vi "PruebaPAI.vi"() -> ()   [LabVIEW 2024]
uses:
  <vilib>/MakerHub/LINX/Public/Peripherals/Digital/Digital Read 1 Chan.vi
  <vilib>/MakerHub/LINX/Public/Peripherals/Digital/Digital Write 1 Chan.vi
  <vilib>/MakerHub/LINX/Public/Peripherals/Digital/Digital Read N Chans.vi
  <vilib>/MakerHub/LINX/Public/Peripherals/Digital/Digital Write N Chans.vi
  <vilib>/MakerHub/LINX/Private/Local IO/LinxDigitalRead.vi
  <vilib>/MakerHub/LINX/Public/Utilities/Check Channel.vi
  <vilib>/MakerHub/LINX/Private/Local IO/LinxDigitalWrite.vi
  <vilib>/MakerHub/LINX/Public/Utilities/Open Serial.vi
  <vilib>/MakerHub/LINX/Private/Utilties/Generate Error.vi
  <vilib>/MakerHub/LINX/LMH-LINX.lvlib
panel:
  in  "Detener":bool
  out "Pin6":dbl
  out "Pin5":dbl
  out "Pin4":dbl
  out "Pin3":dbl
  out "Pin2":dbl
  in  "Puerto Serial":refnum<visa-resource-name>="N/A"
  out "Contenido":dbl
  out "Led 5":bool
  out "Led 4":bool
  out "Led 3":bool
  in  "Secuencia":dbl
  out "Led 2":bool
  out "Led 1":bool
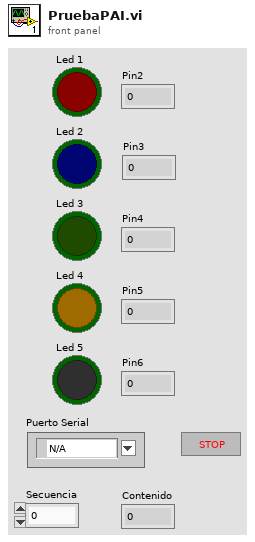
[diagram p1: front panel]
types:
  T1 = typedef "LMH-LINX.lvlib/LINX Ref.ctl" = cluster{"IO":T2, "Interface":T3, "LINX Device Config":T4}
  T2 = typedef "LMH-LINX.lvlib/Platform.ctl" = enum16{"Remote", "Local"}
  T3 = typedef "LMH-LINX.lvlib/Interface.ctl" = enum16{"Serial", "TCP"}
  T4 = typedef "LMH-LINX.lvlib/Device.lvlib/LINX Device Config.ctl" = cluster{"Interface":T3, "COM Port":refnum<visa-resource-name>, "TCP Configuration":T5, "Device Family":u8, "Device ID":u8, "Device Name":string, "TCP Ref":refnum<k5>, "Channels":T6}
  T5 = typedef "LMH-LINX.lvlib/Device.lvlib/TCP Config.ctl" = cluster{"IP Address":string, "Port":u16}
  T6 = typedef "LMH-LINX.lvlib/Channels.ctl" = cluster{"DI":u8[], "DO":u8[], "AI":u8[], "AO":u8[], "PWM":u8[], "QE":u8[], "UART":u8[], "I2C 2":u8[], "SPI":u8[], "CAN":u8[], "Servo":u8[], "AI Ref (V)":dbl, "AI Resolution (Bits)":u8, "AO Ref (V)":dbl, "AO Resolution (Bits)":u8}
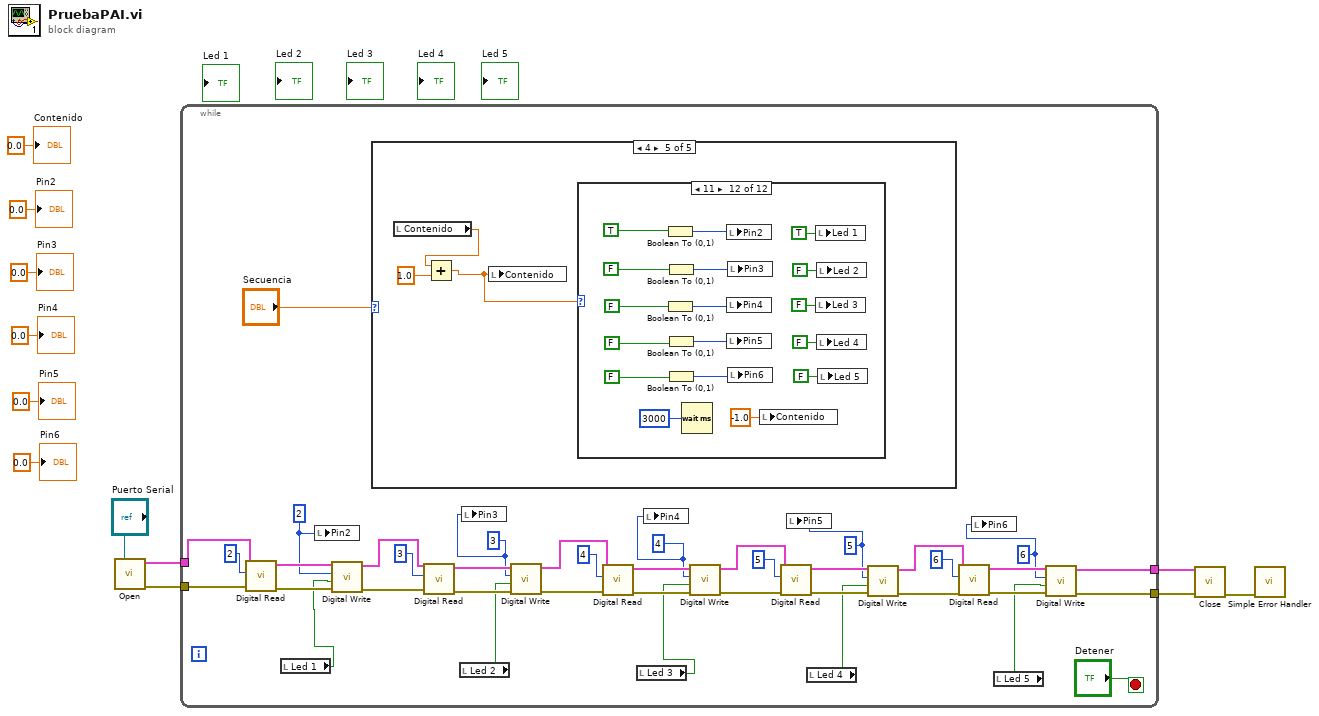
[diagram p0: block diagram]
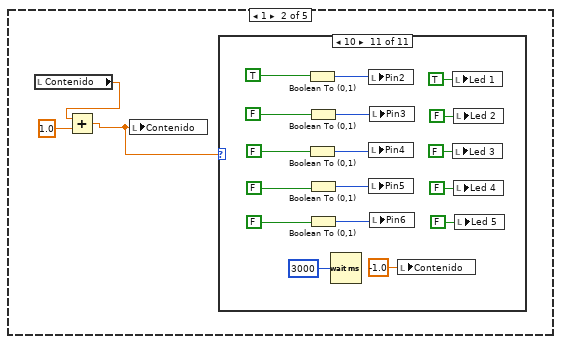
[diagram p3: hidden frame]
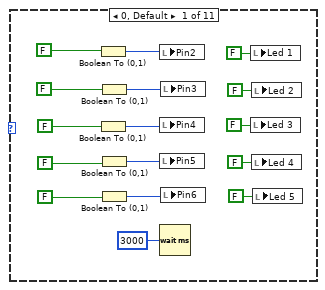
[diagram p4: hidden frame]
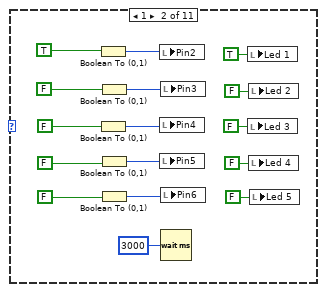
[diagram p5: hidden frame]
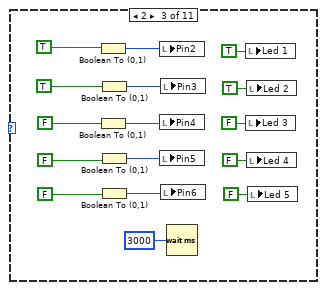
[diagram p6: hidden frame]
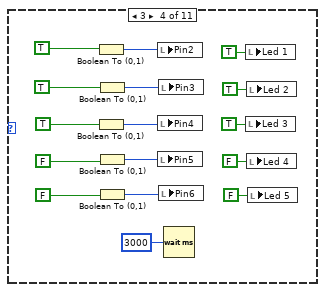
[diagram p7: hidden frame]
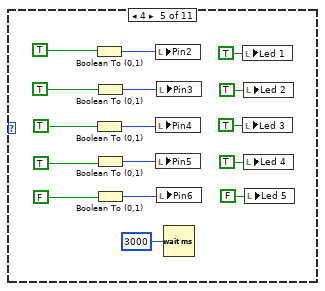
[diagram p8: hidden frame]
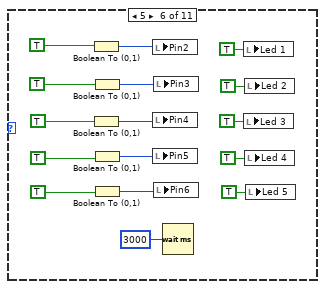
[diagram p9: hidden frame]
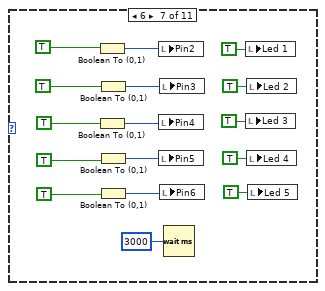
[diagram p10: hidden frame]
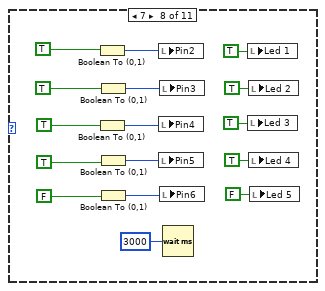
[diagram p11: hidden frame]
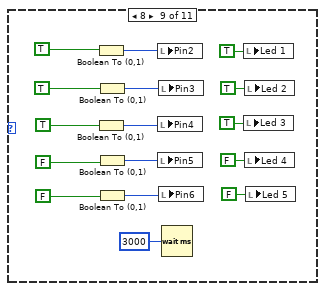
[diagram p12: hidden frame]
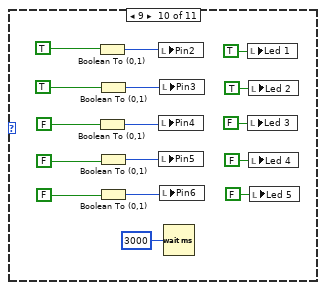
[diagram p13: hidden frame]
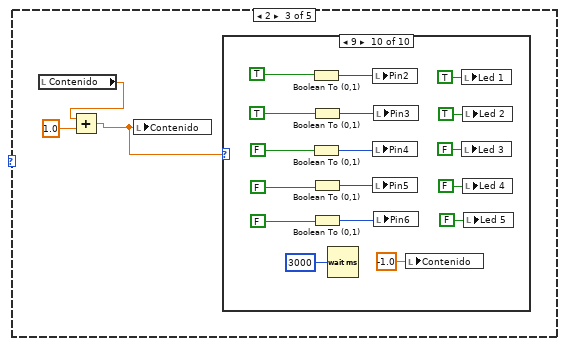
[diagram p14: hidden frame]
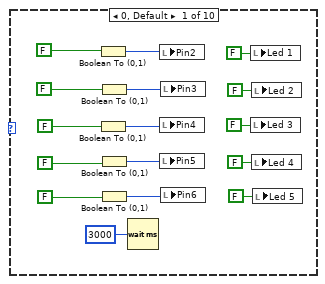
[diagram p15: hidden frame]
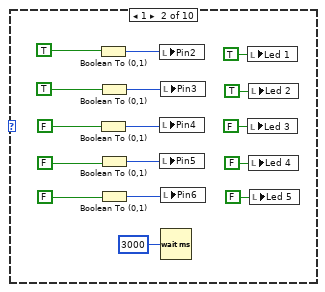
[diagram p16: hidden frame]
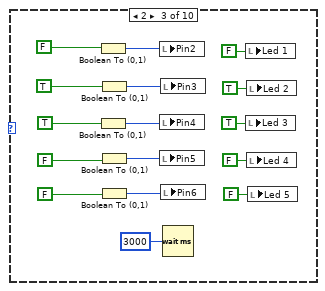
[diagram p17: hidden frame]
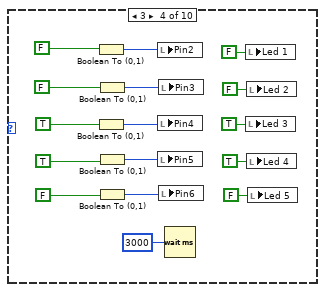
[diagram p18: hidden frame]
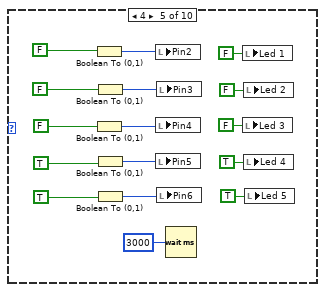
[diagram p19: hidden frame]
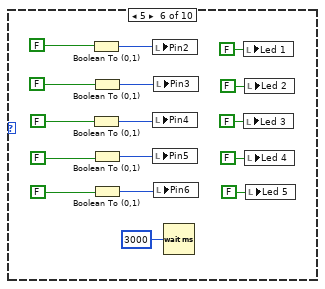
[diagram p20: hidden frame]
diagram:
  n1 = call-poly <vilib>:"Open.vi"("Serial Port"="Puerto Serial") -> ("Error Out"=w1:errorcluster, "LINX Resource"=w2:T1)  [unwired: 8 in, 1 out]
  n2 = while {
    tunnel: [w18] -> w4
    tunnel: [w17] -> w3
    tunnel: w2 -> [w16]
    tunnel: w1 -> [w15]
    stop <- "Detener" stop-if-true
    w19 = u8 6 ("DO Channel")
    w22 = u8 5 ("DO Channel")
    w23 = u8 4 ("DO Channel")
    w28 = u8 3 ("DO Channel")
    w26 = u8 2 ("DO Channel")
    n3 = call-poly <vilib>:"Digital Read.vi"("Error In"=w15, "DI Channel"=u8 2, "LINX Resource"=w16) -> ("Error Out"=w37:errorcluster, "LINX Resource"=w46:T1)  [unwired: 6 in, 1 out]
    n4 = local read "Led 1"() -> (w27:bool)
    n5 = local write "Pin2"(w26) -> ()
    n6 = call-poly <vilib>:"Digital Write.vi"("Error In"=w37, "Output Value"=w27, "DO Channel"=w26, "LINX Resource"=w46) -> ("Error Out"=w36:errorcluster, "LINX Resource"=w45:T1)  [unwired: 6 in]
    n7 = case shown="4" "Secuencia" {
      frame 0, Default {
      }
      frame 1 {
        n8 = local read "Contenido"() -> (w53:dbl)
        n9 = Add(x=w53, y=1.0) -> (x+y=w52:dbl)
        n10 = local write "Contenido"(w52) -> ()
        n11 = case shown="10" w52 {
          frame 0, Default {
            n12 = Boolean To (0,1)(Boolean=FALSE) -> (0, 1=w70:i16)
            n13 = Boolean To (0,1)(Boolean=FALSE) -> (0, 1=w68:i16)
            n14 = Boolean To (0,1)(Boolean=FALSE) -> (0, 1=w69:i16)
            n15 = Boolean To (0,1)(Boolean=FALSE) -> (0, 1=w67:i16)
            n16 = Boolean To (0,1)(Boolean=FALSE) -> (0, 1=w66:i16)
            n17 = local write "Pin2"(w70) -> ()
            n18 = local write "Pin4"(w68) -> ()
            n19 = local write "Pin5"(w67) -> ()
            n20 = Wait (ms)(milliseconds to wait=u32 3000 ("millisecond timer value")) -> ()  [unwired: 1 out]
            n21 = local write "Pin3"(w69) -> ()
            n22 = local write "Pin6"(w66) -> ()
            n23 = local write "Led 1"(FALSE ("Led 1")) -> ()
            n24 = local write "Led 3"(FALSE ("Led 3")) -> ()
            n25 = local write "Led 2"(FALSE ("Led 2")) -> ()
            n26 = local write "Led 4"(FALSE ("Led 4")) -> ()
            n27 = local write "Led 5"(FALSE ("Led 5")) -> ()
          }
          frame 1 {
            n28 = Boolean To (0,1)(Boolean=TRUE) -> (0, 1=w85:i16)
            n29 = Boolean To (0,1)(Boolean=FALSE) -> (0, 1=w81:i16)
            n30 = Boolean To (0,1)(Boolean=FALSE) -> (0, 1=w83:i16)
            n31 = Boolean To (0,1)(Boolean=FALSE) -> (0, 1=w79:i16)
            n32 = Boolean To (0,1)(Boolean=FALSE) -> (0, 1=w77:i16)
            n33 = local write "Pin2"(w85) -> ()
            n34 = local write "Pin4"(w81) -> ()
            n35 = local write "Pin5"(w79) -> ()
            n36 = local write "Pin3"(w83) -> ()
            n37 = local write "Pin6"(w77) -> ()
            n38 = Wait (ms)(milliseconds to wait=u32 3000 ("millisecond timer value")) -> ()  [unwired: 1 out]
            n39 = local write "Led 1"(TRUE ("Led 1")) -> ()
            n40 = local write "Led 3"(FALSE ("Led 3")) -> ()
            n41 = local write "Led 2"(FALSE ("Led 2")) -> ()
            n42 = local write "Led 4"(FALSE ("Led 4")) -> ()
            n43 = local write "Led 5"(FALSE ("Led 5")) -> ()
          }
          frame 2 {
            n44 = Boolean To (0,1)(Boolean=TRUE) -> (0, 1=w102:i16)
            n45 = Boolean To (0,1)(Boolean=FALSE) -> (0, 1=w100:i16)
            n46 = Boolean To (0,1)(Boolean=TRUE) -> (0, 1=w101:i16)
            n47 = Boolean To (0,1)(Boolean=FALSE) -> (0, 1=w99:i16)
            n48 = Boolean To (0,1)(Boolean=FALSE) -> (0, 1=w98:i16)
            n49 = local write "Pin2"(w102) -> ()
            n50 = local write "Pin4"(w100) -> ()
            n51 = local write "Pin5"(w99) -> ()
            n52 = local write "Pin3"(w101) -> ()
            n53 = local write "Pin6"(w98) -> ()
            n54 = Wait (ms)(milliseconds to wait=u32 3000 ("millisecond timer value")) -> ()  [unwired: 1 out]
            n55 = local write "Led 1"(TRUE ("Led 1")) -> ()
            n56 = local write "Led 3"(FALSE ("Led 3")) -> ()
            n57 = local write "Led 2"(TRUE ("Led 2")) -> ()
            n58 = local write "Led 4"(FALSE ("Led 4")) -> ()
            n59 = local write "Led 5"(FALSE ("Led 5")) -> ()
          }
          frame 3 {
            n60 = Boolean To (0,1)(Boolean=TRUE) -> (0, 1=w118:i16)
            n61 = Boolean To (0,1)(Boolean=TRUE) -> (0, 1=w116:i16)
            n62 = Boolean To (0,1)(Boolean=TRUE) -> (0, 1=w117:i16)
            n63 = Boolean To (0,1)(Boolean=FALSE) -> (0, 1=w115:i16)
            n64 = Boolean To (0,1)(Boolean=FALSE) -> (0, 1=w114:i16)
            n65 = local write "Pin2"(w118) -> ()
            n66 = local write "Pin4"(w116) -> ()
            n67 = local write "Pin5"(w115) -> ()
            n68 = local write "Pin3"(w117) -> ()
            n69 = local write "Pin6"(w114) -> ()
            n70 = Wait (ms)(milliseconds to wait=u32 3000 ("millisecond timer value")) -> ()  [unwired: 1 out]
            n71 = local write "Led 1"(TRUE ("Led 1")) -> ()
            n72 = local write "Led 3"(TRUE ("Led 3")) -> ()
            n73 = local write "Led 2"(TRUE ("Led 2")) -> ()
            n74 = local write "Led 4"(FALSE ("Led 4")) -> ()
            n75 = local write "Led 5"(FALSE ("Led 5")) -> ()
          }
          frame 4 {
            n76 = Boolean To (0,1)(Boolean=TRUE) -> (0, 1=w134:i16)
            n77 = Boolean To (0,1)(Boolean=TRUE) -> (0, 1=w132:i16)
            n78 = Boolean To (0,1)(Boolean=TRUE) -> (0, 1=w133:i16)
            n79 = Boolean To (0,1)(Boolean=TRUE) -> (0, 1=w131:i16)
            n80 = Boolean To (0,1)(Boolean=FALSE) -> (0, 1=w130:i16)
            n81 = local write "Pin2"(w134) -> ()
            n82 = local write "Pin4"(w132) -> ()
            n83 = local write "Pin5"(w131) -> ()
            n84 = local write "Pin3"(w133) -> ()
            n85 = local write "Pin6"(w130) -> ()
            n86 = Wait (ms)(milliseconds to wait=u32 3000 ("millisecond timer value")) -> ()  [unwired: 1 out]
            n87 = local write "Led 1"(TRUE ("Led 1")) -> ()
            n88 = local write "Led 3"(TRUE ("Led 3")) -> ()
            n89 = local write "Led 2"(TRUE ("Led 2")) -> ()
            n90 = local write "Led 4"(TRUE ("Led 4")) -> ()
            n91 = local write "Led 5"(FALSE ("Led 5")) -> ()
          }
          frame 5 {
            n92 = Boolean To (0,1)(Boolean=TRUE) -> (0, 1=w150:i16)
            n93 = Boolean To (0,1)(Boolean=TRUE) -> (0, 1=w148:i16)
            n94 = Boolean To (0,1)(Boolean=TRUE) -> (0, 1=w149:i16)
            n95 = Boolean To (0,1)(Boolean=TRUE) -> (0, 1=w147:i16)
            n96 = Boolean To (0,1)(Boolean=TRUE) -> (0, 1=w146:i16)
            n97 = local write "Pin2"(w150) -> ()
            n98 = local write "Pin4"(w148) -> ()
            n99 = local write "Pin5"(w147) -> ()
            n100 = local write "Pin3"(w149) -> ()
            n101 = local write "Pin6"(w146) -> ()
            n102 = Wait (ms)(milliseconds to wait=u32 3000 ("millisecond timer value")) -> ()  [unwired: 1 out]
            n103 = local write "Led 1"(TRUE ("Led 1")) -> ()
            n104 = local write "Led 3"(TRUE ("Led 3")) -> ()
            n105 = local write "Led 2"(TRUE ("Led 2")) -> ()
            n106 = local write "Led 4"(TRUE ("Led 4")) -> ()
            n107 = local write "Led 5"(TRUE ("Led 5")) -> ()
          }
          frame 6 {
            n108 = Boolean To (0,1)(Boolean=TRUE) -> (0, 1=w166:i16)
            n109 = Boolean To (0,1)(Boolean=TRUE) -> (0, 1=w164:i16)
            n110 = Boolean To (0,1)(Boolean=TRUE) -> (0, 1=w165:i16)
            n111 = Boolean To (0,1)(Boolean=TRUE) -> (0, 1=w163:i16)
            n112 = Boolean To (0,1)(Boolean=TRUE) -> (0, 1=w162:i16)
            n113 = local write "Pin2"(w166) -> ()
            n114 = local write "Pin4"(w164) -> ()
            n115 = local write "Pin5"(w163) -> ()
            n116 = local write "Pin3"(w165) -> ()
            n117 = local write "Pin6"(w162) -> ()
            n118 = Wait (ms)(milliseconds to wait=u32 3000 ("millisecond timer value")) -> ()  [unwired: 1 out]
            n119 = local write "Led 1"(TRUE ("Led 1")) -> ()
            n120 = local write "Led 3"(TRUE ("Led 3")) -> ()
            n121 = local write "Led 2"(TRUE ("Led 2")) -> ()
            n122 = local write "Led 4"(TRUE ("Led 4")) -> ()
            n123 = local write "Led 5"(TRUE ("Led 5")) -> ()
          }
          frame 7 {
            n124 = Boolean To (0,1)(Boolean=TRUE) -> (0, 1=w182:i16)
            n125 = Boolean To (0,1)(Boolean=TRUE) -> (0, 1=w180:i16)
            n126 = Boolean To (0,1)(Boolean=TRUE) -> (0, 1=w181:i16)
            n127 = Boolean To (0,1)(Boolean=TRUE) -> (0, 1=w179:i16)
            n128 = Boolean To (0,1)(Boolean=FALSE) -> (0, 1=w178:i16)
            n129 = local write "Pin2"(w182) -> ()
            n130 = local write "Pin4"(w180) -> ()
            n131 = local write "Pin5"(w179) -> ()
            n132 = local write "Pin3"(w181) -> ()
            n133 = local write "Pin6"(w178) -> ()
            n134 = Wait (ms)(milliseconds to wait=u32 3000 ("millisecond timer value")) -> ()  [unwired: 1 out]
            n135 = local write "Led 1"(TRUE ("Led 1")) -> ()
            n136 = local write "Led 3"(TRUE ("Led 3")) -> ()
            n137 = local write "Led 2"(TRUE ("Led 2")) -> ()
            n138 = local write "Led 4"(TRUE ("Led 4")) -> ()
            n139 = local write "Led 5"(FALSE ("Led 5")) -> ()
          }
          frame 8 {
            n140 = Boolean To (0,1)(Boolean=TRUE) -> (0, 1=w198:i16)
            n141 = Boolean To (0,1)(Boolean=TRUE) -> (0, 1=w196:i16)
            n142 = Boolean To (0,1)(Boolean=TRUE) -> (0, 1=w197:i16)
            n143 = Boolean To (0,1)(Boolean=FALSE) -> (0, 1=w195:i16)
            n144 = Boolean To (0,1)(Boolean=FALSE) -> (0, 1=w194:i16)
            n145 = local write "Pin2"(w198) -> ()
            n146 = local write "Pin4"(w196) -> ()
            n147 = local write "Pin5"(w195) -> ()
            n148 = local write "Pin3"(w197) -> ()
            n149 = local write "Pin6"(w194) -> ()
            n150 = Wait (ms)(milliseconds to wait=u32 3000 ("millisecond timer value")) -> ()  [unwired: 1 out]
            n151 = local write "Led 1"(TRUE ("Led 1")) -> ()
            n152 = local write "Led 3"(TRUE ("Led 3")) -> ()
            n153 = local write "Led 2"(TRUE ("Led 2")) -> ()
            n154 = local write "Led 4"(FALSE ("Led 4")) -> ()
            n155 = local write "Led 5"(FALSE ("Led 5")) -> ()
          }
          frame 9 {
            n156 = Boolean To (0,1)(Boolean=TRUE) -> (0, 1=w214:i16)
            n157 = Boolean To (0,1)(Boolean=FALSE) -> (0, 1=w212:i16)
            n158 = Boolean To (0,1)(Boolean=TRUE) -> (0, 1=w213:i16)
            n159 = Boolean To (0,1)(Boolean=FALSE) -> (0, 1=w211:i16)
            n160 = Boolean To (0,1)(Boolean=FALSE) -> (0, 1=w210:i16)
            n161 = local write "Pin2"(w214) -> ()
            n162 = local write "Pin4"(w212) -> ()
            n163 = local write "Pin5"(w211) -> ()
            n164 = local write "Pin3"(w213) -> ()
            n165 = local write "Pin6"(w210) -> ()
            n166 = Wait (ms)(milliseconds to wait=u32 3000 ("millisecond timer value")) -> ()  [unwired: 1 out]
            n167 = local write "Led 1"(TRUE ("Led 1")) -> ()
            n168 = local write "Led 3"(FALSE ("Led 3")) -> ()
            n169 = local write "Led 2"(TRUE ("Led 2")) -> ()
            n170 = local write "Led 4"(FALSE ("Led 4")) -> ()
            n171 = local write "Led 5"(FALSE ("Led 5")) -> ()
          }
          frame 10 {
            n172 = Boolean To (0,1)(Boolean=TRUE) -> (0, 1=w231:i16)
            n173 = Boolean To (0,1)(Boolean=FALSE) -> (0, 1=w229:i16)
            n174 = Boolean To (0,1)(Boolean=FALSE) -> (0, 1=w230:i16)
            n175 = Boolean To (0,1)(Boolean=FALSE) -> (0, 1=w228:i16)
            n176 = Boolean To (0,1)(Boolean=FALSE) -> (0, 1=w227:i16)
            n177 = Wait (ms)(milliseconds to wait=u32 3000 ("millisecond timer value")) -> ()  [unwired: 1 out]
            n178 = local write "Pin2"(w231) -> ()
            n179 = local write "Pin4"(w229) -> ()
            n180 = local write "Pin5"(w228) -> ()
            n181 = local write "Pin3"(w230) -> ()
            n182 = local write "Pin6"(w227) -> ()
            n183 = local write "Contenido"(-1.0 ("Contenido")) -> ()
            n184 = local write "Led 1"(TRUE ("Led 1")) -> ()
            n185 = local write "Led 3"(FALSE ("Led 3")) -> ()
            n186 = local write "Led 2"(FALSE ("Led 2")) -> ()
            n187 = local write "Led 4"(FALSE ("Led 4")) -> ()
            n188 = local write "Led 5"(FALSE ("Led 5")) -> ()
          }
        }
      }
      frame 2 {
        n189 = local read "Contenido"() -> (w234:dbl)
        n190 = Add(x=w234, y=1.0) -> (x+y=w233:dbl)
        n191 = local write "Contenido"(w233) -> ()
        n192 = case shown="9" w233 {
          frame 0, Default {
            n193 = Boolean To (0,1)(Boolean=FALSE) -> (0, 1=w250:i16)
            n194 = Boolean To (0,1)(Boolean=FALSE) -> (0, 1=w248:i16)
            n195 = Boolean To (0,1)(Boolean=FALSE) -> (0, 1=w249:i16)
            n196 = Boolean To (0,1)(Boolean=FALSE) -> (0, 1=w247:i16)
            n197 = Boolean To (0,1)(Boolean=FALSE) -> (0, 1=w246:i16)
            n198 = Wait (ms)(milliseconds to wait=u32 3000 ("millisecond timer value")) -> ()  [unwired: 1 out]
            n199 = local write "Pin2"(w250) -> ()
            n200 = local write "Pin4"(w248) -> ()
            n201 = local write "Pin5"(w247) -> ()
            n202 = local write "Pin3"(w249) -> ()
            n203 = local write "Pin6"(w246) -> ()
            n204 = local write "Led 1"(FALSE ("Led 1")) -> ()
            n205 = local write "Led 3"(FALSE ("Led 3")) -> ()
            n206 = local write "Led 2"(FALSE ("Led 2")) -> ()
            n207 = local write "Led 4"(FALSE ("Led 4")) -> ()
            n208 = local write "Led 5"(FALSE ("Led 5")) -> ()
          }
          frame 1 {
            n209 = Boolean To (0,1)(Boolean=TRUE) -> (0, 1=w265:i16)
            n210 = Boolean To (0,1)(Boolean=FALSE) -> (0, 1=w261:i16)
            n211 = Boolean To (0,1)(Boolean=TRUE) -> (0, 1=w263:i16)
            n212 = Boolean To (0,1)(Boolean=FALSE) -> (0, 1=w259:i16)
            n213 = Boolean To (0,1)(Boolean=FALSE) -> (0, 1=w257:i16)
            n214 = local write "Pin2"(w265) -> ()
            n215 = local write "Pin4"(w261) -> ()
            n216 = local write "Pin5"(w259) -> ()
            n217 = local write "Pin3"(w263) -> ()
            n218 = local write "Pin6"(w257) -> ()
            n219 = Wait (ms)(milliseconds to wait=u32 3000 ("millisecond timer value")) -> ()  [unwired: 1 out]
            n220 = local write "Led 1"(TRUE ("Led 1")) -> ()
            n221 = local write "Led 3"(FALSE ("Led 3")) -> ()
            n222 = local write "Led 2"(TRUE ("Led 2")) -> ()
            n223 = local write "Led 4"(FALSE ("Led 4")) -> ()
            n224 = local write "Led 5"(FALSE ("Led 5")) -> ()
          }
          frame 2 {
            n225 = Boolean To (0,1)(Boolean=FALSE) -> (0, 1=w282:i16)
            n226 = Boolean To (0,1)(Boolean=TRUE) -> (0, 1=w280:i16)
            n227 = Boolean To (0,1)(Boolean=TRUE) -> (0, 1=w281:i16)
            n228 = Boolean To (0,1)(Boolean=FALSE) -> (0, 1=w279:i16)
            n229 = Boolean To (0,1)(Boolean=FALSE) -> (0, 1=w278:i16)
            n230 = local write "Pin2"(w282) -> ()
            n231 = local write "Pin4"(w280) -> ()
            n232 = local write "Pin5"(w279) -> ()
            n233 = local write "Pin3"(w281) -> ()
            n234 = local write "Pin6"(w278) -> ()
            n235 = Wait (ms)(milliseconds to wait=u32 3000 ("millisecond timer value")) -> ()  [unwired: 1 out]
            n236 = local write "Led 1"(FALSE ("Led 1")) -> ()
            n237 = local write "Led 3"(TRUE ("Led 3")) -> ()
            n238 = local write "Led 2"(TRUE ("Led 2")) -> ()
            n239 = local write "Led 4"(FALSE ("Led 4")) -> ()
            n240 = local write "Led 5"(FALSE ("Led 5")) -> ()
          }
          frame 3 {
            n241 = Boolean To (0,1)(Boolean=FALSE) -> (0, 1=w298:i16)
            n242 = Boolean To (0,1)(Boolean=TRUE) -> (0, 1=w296:i16)
            n243 = Boolean To (0,1)(Boolean=FALSE) -> (0, 1=w297:i16)
            n244 = Boolean To (0,1)(Boolean=TRUE) -> (0, 1=w295:i16)
            n245 = Boolean To (0,1)(Boolean=FALSE) -> (0, 1=w294:i16)
            n246 = local write "Pin2"(w298) -> ()
            n247 = local write "Pin4"(w296) -> ()
            n248 = local write "Pin5"(w295) -> ()
            n249 = local write "Pin3"(w297) -> ()
            n250 = local write "Pin6"(w294) -> ()
            n251 = Wait (ms)(milliseconds to wait=u32 3000 ("millisecond timer value")) -> ()  [unwired: 1 out]
            n252 = local write "Led 1"(FALSE ("Led 1")) -> ()
            n253 = local write "Led 3"(TRUE ("Led 3")) -> ()
            n254 = local write "Led 2"(FALSE ("Led 2")) -> ()
            n255 = local write "Led 4"(TRUE ("Led 4")) -> ()
            n256 = local write "Led 5"(FALSE ("Led 5")) -> ()
          }
          frame 4 {
            n257 = Boolean To (0,1)(Boolean=FALSE) -> (0, 1=w314:i16)
            n258 = Boolean To (0,1)(Boolean=FALSE) -> (0, 1=w312:i16)
            n259 = Boolean To (0,1)(Boolean=FALSE) -> (0, 1=w313:i16)
            n260 = Boolean To (0,1)(Boolean=TRUE) -> (0, 1=w311:i16)
            n261 = Boolean To (0,1)(Boolean=TRUE) -> (0, 1=w310:i16)
            n262 = local write "Pin2"(w314) -> ()
            n263 = local write "Pin4"(w312) -> ()
            n264 = local write "Pin5"(w311) -> ()
            n265 = local write "Pin3"(w313) -> ()
            n266 = local write "Pin6"(w310) -> ()
            n267 = Wait (ms)(milliseconds to wait=u32 3000 ("millisecond timer value")) -> ()  [unwired: 1 out]
            n268 = local write "Led 1"(FALSE ("Led 1")) -> ()
            n269 = local write "Led 3"(FALSE ("Led 3")) -> ()
            n270 = local write "Led 2"(FALSE ("Led 2")) -> ()
            n271 = local write "Led 4"(TRUE ("Led 4")) -> ()
            n272 = local write "Led 5"(TRUE ("Led 5")) -> ()
          }
          frame 5 {
            n273 = Boolean To (0,1)(Boolean=FALSE) -> (0, 1=w330:i16)
            n274 = Boolean To (0,1)(Boolean=FALSE) -> (0, 1=w328:i16)
            n275 = Boolean To (0,1)(Boolean=FALSE) -> (0, 1=w329:i16)
            n276 = Boolean To (0,1)(Boolean=FALSE) -> (0, 1=w327:i16)
            n277 = Boolean To (0,1)(Boolean=FALSE) -> (0, 1=w326:i16)
            n278 = local write "Pin2"(w330) -> ()
            n279 = local write "Pin4"(w328) -> ()
            n280 = local write "Pin5"(w327) -> ()
            n281 = local write "Pin3"(w329) -> ()
            n282 = local write "Pin6"(w326) -> ()
            n283 = Wait (ms)(milliseconds to wait=u32 3000 ("millisecond timer value")) -> ()  [unwired: 1 out]
            n284 = local write "Led 1"(FALSE ("Led 1")) -> ()
            n285 = local write "Led 3"(FALSE ("Led 3")) -> ()
            n286 = local write "Led 2"(FALSE ("Led 2")) -> ()
            n287 = local write "Led 4"(FALSE ("Led 4")) -> ()
            n288 = local write "Led 5"(FALSE ("Led 5")) -> ()
          }
          frame 6 {
            n289 = Boolean To (0,1)(Boolean=FALSE) -> (0, 1=w346:i16)
            n290 = Boolean To (0,1)(Boolean=FALSE) -> (0, 1=w344:i16)
            n291 = Boolean To (0,1)(Boolean=FALSE) -> (0, 1=w345:i16)
            n292 = Boolean To (0,1)(Boolean=TRUE) -> (0, 1=w343:i16)
            n293 = Boolean To (0,1)(Boolean=TRUE) -> (0, 1=w342:i16)
            n294 = local write "Pin2"(w346) -> ()
            n295 = local write "Pin4"(w344) -> ()
            n296 = local write "Pin5"(w343) -> ()
            n297 = local write "Pin3"(w345) -> ()
            n298 = local write "Pin6"(w342) -> ()
            n299 = Wait (ms)(milliseconds to wait=u32 3000 ("millisecond timer value")) -> ()  [unwired: 1 out]
            n300 = local write "Led 1"(FALSE ("Led 1")) -> ()
            n301 = local write "Led 3"(FALSE ("Led 3")) -> ()
            n302 = local write "Led 2"(FALSE ("Led 2")) -> ()
            n303 = local write "Led 4"(TRUE ("Led 4")) -> ()
            n304 = local write "Led 5"(TRUE ("Led 5")) -> ()
          }
          frame 7 {
            n305 = Boolean To (0,1)(Boolean=FALSE) -> (0, 1=w362:i16)
            n306 = Boolean To (0,1)(Boolean=TRUE) -> (0, 1=w360:i16)
            n307 = Boolean To (0,1)(Boolean=FALSE) -> (0, 1=w361:i16)
            n308 = Boolean To (0,1)(Boolean=TRUE) -> (0, 1=w359:i16)
            n309 = Boolean To (0,1)(Boolean=FALSE) -> (0, 1=w358:i16)
            n310 = local write "Pin2"(w362) -> ()
            n311 = local write "Pin4"(w360) -> ()
            n312 = local write "Pin5"(w359) -> ()
            n313 = local write "Pin3"(w361) -> ()
            n314 = local write "Pin6"(w358) -> ()
            n315 = Wait (ms)(milliseconds to wait=u32 3000 ("millisecond timer value")) -> ()  [unwired: 1 out]
            n316 = local write "Led 1"(FALSE ("Led 1")) -> ()
            n317 = local write "Led 3"(TRUE ("Led 3")) -> ()
            n318 = local write "Led 2"(FALSE ("Led 2")) -> ()
            n319 = local write "Led 4"(TRUE ("Led 4")) -> ()
            n320 = local write "Led 5"(FALSE ("Led 5")) -> ()
          }
          frame 8 {
            n321 = Boolean To (0,1)(Boolean=FALSE) -> (0, 1=w378:i16)
            n322 = Boolean To (0,1)(Boolean=TRUE) -> (0, 1=w376:i16)
            n323 = Boolean To (0,1)(Boolean=TRUE) -> (0, 1=w377:i16)
            n324 = Boolean To (0,1)(Boolean=FALSE) -> (0, 1=w375:i16)
            n325 = Boolean To (0,1)(Boolean=FALSE) -> (0, 1=w374:i16)
            n326 = local write "Pin2"(w378) -> ()
            n327 = local write "Pin4"(w376) -> ()
            n328 = local write "Pin5"(w375) -> ()
            n329 = local write "Pin3"(w377) -> ()
            n330 = local write "Pin6"(w374) -> ()
            n331 = Wait (ms)(milliseconds to wait=u32 3000 ("millisecond timer value")) -> ()  [unwired: 1 out]
            n332 = local write "Led 1"(FALSE ("Led 1")) -> ()
            n333 = local write "Led 3"(TRUE ("Led 3")) -> ()
            n334 = local write "Led 2"(TRUE ("Led 2")) -> ()
            n335 = local write "Led 4"(FALSE ("Led 4")) -> ()
            n336 = local write "Led 5"(FALSE ("Led 5")) -> ()
          }
          frame 9 {
            n337 = Boolean To (0,1)(Boolean=TRUE) -> (0, 1=w395:i16)
            n338 = Boolean To (0,1)(Boolean=FALSE) -> (0, 1=w393:i16)
            n339 = Boolean To (0,1)(Boolean=TRUE) -> (0, 1=w394:i16)
            n340 = Boolean To (0,1)(Boolean=FALSE) -> (0, 1=w392:i16)
            n341 = Boolean To (0,1)(Boolean=FALSE) -> (0, 1=w391:i16)
            n342 = Wait (ms)(milliseconds to wait=u32 3000 ("millisecond timer value")) -> ()  [unwired: 1 out]
            n343 = local write "Pin2"(w395) -> ()
            n344 = local write "Pin4"(w393) -> ()
            n345 = local write "Pin5"(w392) -> ()
            n346 = local write "Pin3"(w394) -> ()
            n347 = local write "Pin6"(w391) -> ()
            n348 = local write "Contenido"(-1.0 ("Contenido")) -> ()
            n349 = local write "Led 1"(TRUE ("Led 1")) -> ()
            n350 = local write "Led 3"(FALSE ("Led 3")) -> ()
            n351 = local write "Led 2"(TRUE ("Led 2")) -> ()
            n352 = local write "Led 4"(FALSE ("Led 4")) -> ()
            n353 = local write "Led 5"(FALSE ("Led 5")) -> ()
          }
        }
      }
      frame 3 {
        n354 = local read "Contenido"() -> (w398:dbl)
        n355 = Add(x=w398, y=1.0) -> (x+y=w397:dbl)
        n356 = local write "Contenido"(w397) -> ()
        n357 = case shown="0, Default" w397 {
          frame 0, Default {
            n358 = Boolean To (0,1)(Boolean=FALSE) -> (0, 1=w414:i16)
            n359 = Boolean To (0,1)(Boolean=FALSE) -> (0, 1=w412:i16)
            n360 = Boolean To (0,1)(Boolean=FALSE) -> (0, 1=w413:i16)
            n361 = Boolean To (0,1)(Boolean=FALSE) -> (0, 1=w411:i16)
            n362 = Boolean To (0,1)(Boolean=FALSE) -> (0, 1=w410:i16)
            n363 = local write "Pin2"(w414) -> ()
            n364 = local write "Pin4"(w412) -> ()
            n365 = local write "Pin5"(w411) -> ()
            n366 = local write "Pin3"(w413) -> ()
            n367 = local write "Pin6"(w410) -> ()
            n368 = Wait (ms)(milliseconds to wait=u32 3000 ("millisecond timer value")) -> ()  [unwired: 1 out]
            n369 = local write "Led 1"(FALSE ("Led 1")) -> ()
            n370 = local write "Led 3"(FALSE ("Led 3")) -> ()
            n371 = local write "Led 2"(FALSE ("Led 2")) -> ()
            n372 = local write "Led 4"(FALSE ("Led 4")) -> ()
            n373 = local write "Led 5"(FALSE ("Led 5")) -> ()
          }
          frame 1 {
            n374 = Boolean To (0,1)(Boolean=TRUE) -> (0, 1=w429:i16)
            n375 = Boolean To (0,1)(Boolean=FALSE) -> (0, 1=w425:i16)
            n376 = Boolean To (0,1)(Boolean=FALSE) -> (0, 1=w427:i16)
            n377 = Boolean To (0,1)(Boolean=FALSE) -> (0, 1=w423:i16)
            n378 = Boolean To (0,1)(Boolean=TRUE) -> (0, 1=w421:i16)
            n379 = local write "Pin2"(w429) -> ()
            n380 = local write "Pin4"(w425) -> ()
            n381 = local write "Pin5"(w423) -> ()
            n382 = local write "Pin3"(w427) -> ()
            n383 = local write "Pin6"(w421) -> ()
            n384 = Wait (ms)(milliseconds to wait=u32 3000 ("millisecond timer value")) -> ()  [unwired: 1 out]
            n385 = local write "Led 1"(TRUE ("Led 1")) -> ()
            n386 = local write "Led 3"(FALSE ("Led 3")) -> ()
            n387 = local write "Led 2"(FALSE ("Led 2")) -> ()
            n388 = local write "Led 4"(FALSE ("Led 4")) -> ()
            n389 = local write "Led 5"(TRUE ("Led 5")) -> ()
          }
          frame 2 {
            n390 = Boolean To (0,1)(Boolean=FALSE) -> (0, 1=w446:i16)
            n391 = Boolean To (0,1)(Boolean=FALSE) -> (0, 1=w444:i16)
            n392 = Boolean To (0,1)(Boolean=TRUE) -> (0, 1=w445:i16)
            n393 = Boolean To (0,1)(Boolean=TRUE) -> (0, 1=w443:i16)
            n394 = Boolean To (0,1)(Boolean=FALSE) -> (0, 1=w442:i16)
            n395 = local write "Pin2"(w446) -> ()
            n396 = local write "Pin4"(w444) -> ()
            n397 = local write "Pin5"(w443) -> ()
            n398 = local write "Pin3"(w445) -> ()
            n399 = local write "Pin6"(w442) -> ()
            n400 = Wait (ms)(milliseconds to wait=u32 3000 ("millisecond timer value")) -> ()  [unwired: 1 out]
            n401 = local write "Led 1"(FALSE ("Led 1")) -> ()
            n402 = local write "Led 3"(FALSE ("Led 3")) -> ()
            n403 = local write "Led 2"(TRUE ("Led 2")) -> ()
            n404 = local write "Led 4"(TRUE ("Led 4")) -> ()
            n405 = local write "Led 5"(FALSE ("Led 5")) -> ()
          }
          frame 3 {
            n406 = Boolean To (0,1)(Boolean=TRUE) -> (0, 1=w462:i16)
            n407 = Boolean To (0,1)(Boolean=TRUE) -> (0, 1=w460:i16)
            n408 = Boolean To (0,1)(Boolean=FALSE) -> (0, 1=w461:i16)
            n409 = Boolean To (0,1)(Boolean=FALSE) -> (0, 1=w459:i16)
            n410 = Boolean To (0,1)(Boolean=FALSE) -> (0, 1=w458:i16)
            n411 = local write "Pin2"(w462) -> ()
            n412 = local write "Pin4"(w460) -> ()
            n413 = local write "Pin5"(w459) -> ()
            n414 = local write "Pin3"(w461) -> ()
            n415 = local write "Pin6"(w458) -> ()
            n416 = Wait (ms)(milliseconds to wait=u32 3000 ("millisecond timer value")) -> ()  [unwired: 1 out]
            n417 = local write "Led 1"(TRUE ("Led 1")) -> ()
            n418 = local write "Led 3"(TRUE ("Led 3")) -> ()
            n419 = local write "Led 2"(FALSE ("Led 2")) -> ()
            n420 = local write "Led 4"(FALSE ("Led 4")) -> ()
            n421 = local write "Led 5"(FALSE ("Led 5")) -> ()
          }
          frame 4 {
            n422 = Boolean To (0,1)(Boolean=FALSE) -> (0, 1=w478:i16)
            n423 = Boolean To (0,1)(Boolean=FALSE) -> (0, 1=w476:i16)
            n424 = Boolean To (0,1)(Boolean=TRUE) -> (0, 1=w477:i16)
            n425 = Boolean To (0,1)(Boolean=TRUE) -> (0, 1=w475:i16)
            n426 = Boolean To (0,1)(Boolean=FALSE) -> (0, 1=w474:i16)
            n427 = local write "Pin2"(w478) -> ()
            n428 = local write "Pin4"(w476) -> ()
            n429 = local write "Pin5"(w475) -> ()
            n430 = local write "Pin3"(w477) -> ()
            n431 = local write "Pin6"(w474) -> ()
            n432 = Wait (ms)(milliseconds to wait=u32 3000 ("millisecond timer value")) -> ()  [unwired: 1 out]
            n433 = local write "Led 1"(FALSE ("Led 1")) -> ()
            n434 = local write "Led 3"(FALSE ("Led 3")) -> ()
            n435 = local write "Led 2"(TRUE ("Led 2")) -> ()
            n436 = local write "Led 4"(TRUE ("Led 4")) -> ()
            n437 = local write "Led 5"(FALSE ("Led 5")) -> ()
          }
          frame 5 {
            n438 = Boolean To (0,1)(Boolean=FALSE) -> (0, 1=w494:i16)
            n439 = Boolean To (0,1)(Boolean=TRUE) -> (0, 1=w492:i16)
            n440 = Boolean To (0,1)(Boolean=FALSE) -> (0, 1=w493:i16)
            n441 = Boolean To (0,1)(Boolean=FALSE) -> (0, 1=w491:i16)
            n442 = Boolean To (0,1)(Boolean=TRUE) -> (0, 1=w490:i16)
            n443 = local write "Pin2"(w494) -> ()
            n444 = local write "Pin4"(w492) -> ()
            n445 = local write "Pin5"(w491) -> ()
            n446 = local write "Pin3"(w493) -> ()
            n447 = local write "Pin6"(w490) -> ()
            n448 = Wait (ms)(milliseconds to wait=u32 3000 ("millisecond timer value")) -> ()  [unwired: 1 out]
            n449 = local write "Led 1"(FALSE ("Led 1")) -> ()
            n450 = local write "Led 3"(TRUE ("Led 3")) -> ()
            n451 = local write "Led 2"(FALSE ("Led 2")) -> ()
            n452 = local write "Led 4"(FALSE ("Led 4")) -> ()
            n453 = local write "Led 5"(TRUE ("Led 5")) -> ()
          }
          frame 6 {
            n454 = Boolean To (0,1)(Boolean=FALSE) -> (0, 1=w510:i16)
            n455 = Boolean To (0,1)(Boolean=FALSE) -> (0, 1=w508:i16)
            n456 = Boolean To (0,1)(Boolean=FALSE) -> (0, 1=w509:i16)
            n457 = Boolean To (0,1)(Boolean=FALSE) -> (0, 1=w507:i16)
            n458 = Boolean To (0,1)(Boolean=FALSE) -> (0, 1=w506:i16)
            n459 = local write "Pin2"(w510) -> ()
            n460 = local write "Pin4"(w508) -> ()
            n461 = local write "Pin5"(w507) -> ()
            n462 = local write "Pin3"(w509) -> ()
            n463 = local write "Pin6"(w506) -> ()
            n464 = Wait (ms)(milliseconds to wait=u32 3000 ("millisecond timer value")) -> ()  [unwired: 1 out]
            n465 = local write "Led 1"(FALSE ("Led 1")) -> ()
            n466 = local write "Led 3"(FALSE ("Led 3")) -> ()
            n467 = local write "Led 2"(FALSE ("Led 2")) -> ()
            n468 = local write "Led 4"(FALSE ("Led 4")) -> ()
            n469 = local write "Led 5"(FALSE ("Led 5")) -> ()
          }
          frame 7 {
            n470 = Boolean To (0,1)(Boolean=FALSE) -> (0, 1=w526:i16)
            n471 = Boolean To (0,1)(Boolean=TRUE) -> (0, 1=w524:i16)
            n472 = Boolean To (0,1)(Boolean=FALSE) -> (0, 1=w525:i16)
            n473 = Boolean To (0,1)(Boolean=FALSE) -> (0, 1=w523:i16)
            n474 = Boolean To (0,1)(Boolean=TRUE) -> (0, 1=w522:i16)
            n475 = local write "Pin2"(w526) -> ()
            n476 = local write "Pin4"(w524) -> ()
            n477 = local write "Pin5"(w523) -> ()
            n478 = local write "Pin3"(w525) -> ()
            n479 = local write "Pin6"(w522) -> ()
            n480 = Wait (ms)(milliseconds to wait=u32 3000 ("millisecond timer value")) -> ()  [unwired: 1 out]
            n481 = local write "Led 1"(FALSE ("Led 1")) -> ()
            n482 = local write "Led 3"(TRUE ("Led 3")) -> ()
            n483 = local write "Led 2"(FALSE ("Led 2")) -> ()
            n484 = local write "Led 4"(FALSE ("Led 4")) -> ()
            n485 = local write "Led 5"(TRUE ("Led 5")) -> ()
          }
          frame 8 {
            n486 = Boolean To (0,1)(Boolean=FALSE) -> (0, 1=w542:i16)
            n487 = Boolean To (0,1)(Boolean=FALSE) -> (0, 1=w540:i16)
            n488 = Boolean To (0,1)(Boolean=TRUE) -> (0, 1=w541:i16)
            n489 = Boolean To (0,1)(Boolean=TRUE) -> (0, 1=w539:i16)
            n490 = Boolean To (0,1)(Boolean=FALSE) -> (0, 1=w538:i16)
            n491 = local write "Pin2"(w542) -> ()
            n492 = local write "Pin4"(w540) -> ()
            n493 = local write "Pin5"(w539) -> ()
            n494 = local write "Pin3"(w541) -> ()
            n495 = local write "Pin6"(w538) -> ()
            n496 = Wait (ms)(milliseconds to wait=u32 3000 ("millisecond timer value")) -> ()  [unwired: 1 out]
            n497 = local write "Led 1"(FALSE ("Led 1")) -> ()
            n498 = local write "Led 3"(FALSE ("Led 3")) -> ()
            n499 = local write "Led 2"(TRUE ("Led 2")) -> ()
            n500 = local write "Led 4"(TRUE ("Led 4")) -> ()
            n501 = local write "Led 5"(FALSE ("Led 5")) -> ()
          }
          frame 9 {
            n502 = Boolean To (0,1)(Boolean=TRUE) -> (0, 1=w558:i16)
            n503 = Boolean To (0,1)(Boolean=TRUE) -> (0, 1=w556:i16)
            n504 = Boolean To (0,1)(Boolean=FALSE) -> (0, 1=w557:i16)
            n505 = Boolean To (0,1)(Boolean=FALSE) -> (0, 1=w555:i16)
            n506 = Boolean To (0,1)(Boolean=FALSE) -> (0, 1=w554:i16)
            n507 = local write "Pin2"(w558) -> ()
            n508 = local write "Pin4"(w556) -> ()
            n509 = local write "Pin5"(w555) -> ()
            n510 = local write "Pin3"(w557) -> ()
            n511 = local write "Pin6"(w554) -> ()
            n512 = Wait (ms)(milliseconds to wait=u32 3000 ("millisecond timer value")) -> ()  [unwired: 1 out]
            n513 = local write "Led 1"(TRUE ("Led 1")) -> ()
            n514 = local write "Led 3"(TRUE ("Led 3")) -> ()
            n515 = local write "Led 2"(FALSE ("Led 2")) -> ()
            n516 = local write "Led 4"(FALSE ("Led 4")) -> ()
            n517 = local write "Led 5"(FALSE ("Led 5")) -> ()
          }
          frame 10 {
            n518 = Boolean To (0,1)(Boolean=FALSE) -> (0, 1=w574:i16)
            n519 = Boolean To (0,1)(Boolean=FALSE) -> (0, 1=w572:i16)
            n520 = Boolean To (0,1)(Boolean=TRUE) -> (0, 1=w573:i16)
            n521 = Boolean To (0,1)(Boolean=TRUE) -> (0, 1=w571:i16)
            n522 = Boolean To (0,1)(Boolean=FALSE) -> (0, 1=w570:i16)
            n523 = local write "Pin2"(w574) -> ()
            n524 = local write "Pin4"(w572) -> ()
            n525 = local write "Pin5"(w571) -> ()
            n526 = local write "Pin3"(w573) -> ()
            n527 = local write "Pin6"(w570) -> ()
            n528 = Wait (ms)(milliseconds to wait=u32 3000 ("millisecond timer value")) -> ()  [unwired: 1 out]
            n529 = local write "Led 1"(FALSE ("Led 1")) -> ()
            n530 = local write "Led 3"(FALSE ("Led 3")) -> ()
            n531 = local write "Led 2"(TRUE ("Led 2")) -> ()
            n532 = local write "Led 4"(TRUE ("Led 4")) -> ()
            n533 = local write "Led 5"(FALSE ("Led 5")) -> ()
          }
          frame 11 {
            n534 = Boolean To (0,1)(Boolean=TRUE) -> (0, 1=w591:i16)
            n535 = Boolean To (0,1)(Boolean=FALSE) -> (0, 1=w589:i16)
            n536 = Boolean To (0,1)(Boolean=FALSE) -> (0, 1=w590:i16)
            n537 = Boolean To (0,1)(Boolean=FALSE) -> (0, 1=w588:i16)
            n538 = Boolean To (0,1)(Boolean=TRUE) -> (0, 1=w587:i16)
            n539 = Wait (ms)(milliseconds to wait=u32 3000 ("millisecond timer value")) -> ()  [unwired: 1 out]
            n540 = local write "Pin2"(w591) -> ()
            n541 = local write "Pin4"(w589) -> ()
            n542 = local write "Pin5"(w588) -> ()
            n543 = local write "Pin3"(w590) -> ()
            n544 = local write "Pin6"(w587) -> ()
            n545 = local write "Contenido"(-1.0 ("Contenido")) -> ()
            n546 = local write "Led 1"(TRUE ("Led 1")) -> ()
            n547 = local write "Led 3"(FALSE ("Led 3")) -> ()
            n548 = local write "Led 2"(FALSE ("Led 2")) -> ()
            n549 = local write "Led 4"(FALSE ("Led 4")) -> ()
            n550 = local write "Led 5"(TRUE ("Led 5")) -> ()
          }
        }
      }
      frame 4 {
        n551 = local read "Contenido"() -> (w594:dbl)
        n552 = Add(x=w594, y=1.0) -> (x+y=w593:dbl)
        n553 = local write "Contenido"(w593) -> ()
        n554 = case shown="11" w593 {
          frame 0, Default {
            n555 = Boolean To (0,1)(Boolean=FALSE) -> (0, 1=w610:i16)
            n556 = Boolean To (0,1)(Boolean=FALSE) -> (0, 1=w608:i16)
            n557 = Boolean To (0,1)(Boolean=FALSE) -> (0, 1=w609:i16)
            n558 = Boolean To (0,1)(Boolean=FALSE) -> (0, 1=w607:i16)
            n559 = Boolean To (0,1)(Boolean=FALSE) -> (0, 1=w606:i16)
            n560 = local write "Pin2"(w610) -> ()
            n561 = local write "Pin4"(w608) -> ()
            n562 = local write "Pin5"(w607) -> ()
            n563 = local write "Pin3"(w609) -> ()
            n564 = local write "Pin6"(w606) -> ()
            n565 = Wait (ms)(milliseconds to wait=u32 3000 ("millisecond timer value")) -> ()  [unwired: 1 out]
            n566 = local write "Led 1"(FALSE ("Led 1")) -> ()
            n567 = local write "Led 3"(FALSE ("Led 3")) -> ()
            n568 = local write "Led 2"(FALSE ("Led 2")) -> ()
            n569 = local write "Led 4"(FALSE ("Led 4")) -> ()
            n570 = local write "Led 5"(FALSE ("Led 5")) -> ()
          }
          frame 1 {
            n571 = Boolean To (0,1)(Boolean=TRUE) -> (0, 1=w625:i16)
            n572 = Boolean To (0,1)(Boolean=FALSE) -> (0, 1=w621:i16)
            n573 = Boolean To (0,1)(Boolean=FALSE) -> (0, 1=w623:i16)
            n574 = Boolean To (0,1)(Boolean=FALSE) -> (0, 1=w619:i16)
            n575 = Boolean To (0,1)(Boolean=FALSE) -> (0, 1=w617:i16)
            n576 = local write "Pin2"(w625) -> ()
            n577 = local write "Pin4"(w621) -> ()
            n578 = local write "Pin5"(w619) -> ()
            n579 = local write "Pin3"(w623) -> ()
            n580 = local write "Pin6"(w617) -> ()
            n581 = Wait (ms)(milliseconds to wait=u32 3000 ("millisecond timer value")) -> ()  [unwired: 1 out]
            n582 = local write "Led 1"(TRUE ("Led 1")) -> ()
            n583 = local write "Led 3"(FALSE ("Led 3")) -> ()
            n584 = local write "Led 2"(FALSE ("Led 2")) -> ()
            n585 = local write "Led 4"(FALSE ("Led 4")) -> ()
            n586 = local write "Led 5"(FALSE ("Led 5")) -> ()
          }
          frame 2 {
            n587 = Boolean To (0,1)(Boolean=FALSE) -> (0, 1=w642:i16)
            n588 = Boolean To (0,1)(Boolean=FALSE) -> (0, 1=w640:i16)
            n589 = Boolean To (0,1)(Boolean=FALSE) -> (0, 1=w641:i16)
            n590 = Boolean To (0,1)(Boolean=TRUE) -> (0, 1=w639:i16)
            n591 = Boolean To (0,1)(Boolean=FALSE) -> (0, 1=w638:i16)
            n592 = local write "Pin2"(w642) -> ()
            n593 = local write "Pin4"(w640) -> ()
            n594 = local write "Pin5"(w639) -> ()
            n595 = local write "Pin3"(w641) -> ()
            n596 = local write "Pin6"(w638) -> ()
            n597 = Wait (ms)(milliseconds to wait=u32 3000 ("millisecond timer value")) -> ()  [unwired: 1 out]
            n598 = local write "Led 1"(FALSE ("Led 1")) -> ()
            n599 = local write "Led 3"(FALSE ("Led 3")) -> ()
            n600 = local write "Led 2"(FALSE ("Led 2")) -> ()
            n601 = local write "Led 4"(TRUE ("Led 4")) -> ()
            n602 = local write "Led 5"(FALSE ("Led 5")) -> ()
          }
          frame 3 {
            n603 = Boolean To (0,1)(Boolean=FALSE) -> (0, 1=w658:i16)
            n604 = Boolean To (0,1)(Boolean=TRUE) -> (0, 1=w656:i16)
            n605 = Boolean To (0,1)(Boolean=FALSE) -> (0, 1=w657:i16)
            n606 = Boolean To (0,1)(Boolean=FALSE) -> (0, 1=w655:i16)
            n607 = Boolean To (0,1)(Boolean=FALSE) -> (0, 1=w654:i16)
            n608 = local write "Pin2"(w658) -> ()
            n609 = local write "Pin4"(w656) -> ()
            n610 = local write "Pin5"(w655) -> ()
            n611 = local write "Pin3"(w657) -> ()
            n612 = local write "Pin6"(w654) -> ()
            n613 = Wait (ms)(milliseconds to wait=u32 3000 ("millisecond timer value")) -> ()  [unwired: 1 out]
            n614 = local write "Led 1"(FALSE ("Led 1")) -> ()
            n615 = local write "Led 3"(TRUE ("Led 3")) -> ()
            n616 = local write "Led 2"(FALSE ("Led 2")) -> ()
            n617 = local write "Led 4"(FALSE ("Led 4")) -> ()
            n618 = local write "Led 5"(FALSE ("Led 5")) -> ()
          }
          frame 4 {
            n619 = Boolean To (0,1)(Boolean=FALSE) -> (0, 1=w674:i16)
            n620 = Boolean To (0,1)(Boolean=FALSE) -> (0, 1=w672:i16)
            n621 = Boolean To (0,1)(Boolean=TRUE) -> (0, 1=w673:i16)
            n622 = Boolean To (0,1)(Boolean=FALSE) -> (0, 1=w671:i16)
            n623 = Boolean To (0,1)(Boolean=FALSE) -> (0, 1=w670:i16)
            n624 = local write "Pin2"(w674) -> ()
            n625 = local write "Pin4"(w672) -> ()
            n626 = local write "Pin5"(w671) -> ()
            n627 = local write "Pin3"(w673) -> ()
            n628 = local write "Pin6"(w670) -> ()
            n629 = Wait (ms)(milliseconds to wait=u32 3000 ("millisecond timer value")) -> ()  [unwired: 1 out]
            n630 = local write "Led 1"(FALSE ("Led 1")) -> ()
            n631 = local write "Led 3"(FALSE ("Led 3")) -> ()
            n632 = local write "Led 2"(TRUE ("Led 2")) -> ()
            n633 = local write "Led 4"(FALSE ("Led 4")) -> ()
            n634 = local write "Led 5"(FALSE ("Led 5")) -> ()
          }
          frame 5 {
            n635 = Boolean To (0,1)(Boolean=FALSE) -> (0, 1=w690:i16)
            n636 = Boolean To (0,1)(Boolean=FALSE) -> (0, 1=w688:i16)
            n637 = Boolean To (0,1)(Boolean=FALSE) -> (0, 1=w689:i16)
            n638 = Boolean To (0,1)(Boolean=FALSE) -> (0, 1=w687:i16)
            n639 = Boolean To (0,1)(Boolean=TRUE) -> (0, 1=w686:i16)
            n640 = local write "Pin2"(w690) -> ()
            n641 = local write "Pin4"(w688) -> ()
            n642 = local write "Pin5"(w687) -> ()
            n643 = local write "Pin3"(w689) -> ()
            n644 = local write "Pin6"(w686) -> ()
            n645 = Wait (ms)(milliseconds to wait=u32 3000 ("millisecond timer value")) -> ()  [unwired: 1 out]
            n646 = local write "Led 1"(FALSE ("Led 1")) -> ()
            n647 = local write "Led 3"(FALSE ("Led 3")) -> ()
            n648 = local write "Led 2"(FALSE ("Led 2")) -> ()
            n649 = local write "Led 4"(FALSE ("Led 4")) -> ()
            n650 = local write "Led 5"(TRUE ("Led 5")) -> ()
          }
          frame 6 {
            n651 = Boolean To (0,1)(Boolean=FALSE) -> (0, 1=w706:i16)
            n652 = Boolean To (0,1)(Boolean=FALSE) -> (0, 1=w704:i16)
            n653 = Boolean To (0,1)(Boolean=FALSE) -> (0, 1=w705:i16)
            n654 = Boolean To (0,1)(Boolean=FALSE) -> (0, 1=w703:i16)
            n655 = Boolean To (0,1)(Boolean=FALSE) -> (0, 1=w702:i16)
            n656 = local write "Pin2"(w706) -> ()
            n657 = local write "Pin4"(w704) -> ()
            n658 = local write "Pin5"(w703) -> ()
            n659 = local write "Pin3"(w705) -> ()
            n660 = local write "Pin6"(w702) -> ()
            n661 = Wait (ms)(milliseconds to wait=u32 3000 ("millisecond timer value")) -> ()  [unwired: 1 out]
            n662 = local write "Led 1"(FALSE ("Led 1")) -> ()
            n663 = local write "Led 3"(FALSE ("Led 3")) -> ()
            n664 = local write "Led 2"(FALSE ("Led 2")) -> ()
            n665 = local write "Led 4"(FALSE ("Led 4")) -> ()
            n666 = local write "Led 5"(FALSE ("Led 5")) -> ()
          }
          frame 7 {
            n667 = Boolean To (0,1)(Boolean=FALSE) -> (0, 1=w722:i16)
            n668 = Boolean To (0,1)(Boolean=FALSE) -> (0, 1=w720:i16)
            n669 = Boolean To (0,1)(Boolean=FALSE) -> (0, 1=w721:i16)
            n670 = Boolean To (0,1)(Boolean=FALSE) -> (0, 1=w719:i16)
            n671 = Boolean To (0,1)(Boolean=TRUE) -> (0, 1=w718:i16)
            n672 = local write "Pin2"(w722) -> ()
            n673 = local write "Pin4"(w720) -> ()
            n674 = local write "Pin5"(w719) -> ()
            n675 = local write "Pin3"(w721) -> ()
            n676 = local write "Pin6"(w718) -> ()
            n677 = Wait (ms)(milliseconds to wait=u32 3000 ("millisecond timer value")) -> ()  [unwired: 1 out]
            n678 = local write "Led 1"(FALSE ("Led 1")) -> ()
            n679 = local write "Led 3"(FALSE ("Led 3")) -> ()
            n680 = local write "Led 2"(FALSE ("Led 2")) -> ()
            n681 = local write "Led 4"(FALSE ("Led 4")) -> ()
            n682 = local write "Led 5"(TRUE ("Led 5")) -> ()
          }
          frame 8 {
            n683 = Boolean To (0,1)(Boolean=FALSE) -> (0, 1=w738:i16)
            n684 = Boolean To (0,1)(Boolean=TRUE) -> (0, 1=w736:i16)
            n685 = Boolean To (0,1)(Boolean=FALSE) -> (0, 1=w737:i16)
            n686 = Boolean To (0,1)(Boolean=FALSE) -> (0, 1=w735:i16)
            n687 = Boolean To (0,1)(Boolean=FALSE) -> (0, 1=w734:i16)
            n688 = local write "Pin2"(w738) -> ()
            n689 = local write "Pin4"(w736) -> ()
            n690 = local write "Pin5"(w735) -> ()
            n691 = local write "Pin3"(w737) -> ()
            n692 = local write "Pin6"(w734) -> ()
            n693 = Wait (ms)(milliseconds to wait=u32 3000 ("millisecond timer value")) -> ()  [unwired: 1 out]
            n694 = local write "Led 1"(FALSE ("Led 1")) -> ()
            n695 = local write "Led 3"(TRUE ("Led 3")) -> ()
            n696 = local write "Led 2"(FALSE ("Led 2")) -> ()
            n697 = local write "Led 4"(FALSE ("Led 4")) -> ()
            n698 = local write "Led 5"(FALSE ("Led 5")) -> ()
          }
          frame 9 {
            n699 = Boolean To (0,1)(Boolean=FALSE) -> (0, 1=w754:i16)
            n700 = Boolean To (0,1)(Boolean=FALSE) -> (0, 1=w752:i16)
            n701 = Boolean To (0,1)(Boolean=TRUE) -> (0, 1=w753:i16)
            n702 = Boolean To (0,1)(Boolean=FALSE) -> (0, 1=w751:i16)
            n703 = Boolean To (0,1)(Boolean=FALSE) -> (0, 1=w750:i16)
            n704 = local write "Pin2"(w754) -> ()
            n705 = local write "Pin4"(w752) -> ()
            n706 = local write "Pin5"(w751) -> ()
            n707 = local write "Pin3"(w753) -> ()
            n708 = local write "Pin6"(w750) -> ()
            n709 = Wait (ms)(milliseconds to wait=u32 3000 ("millisecond timer value")) -> ()  [unwired: 1 out]
            n710 = local write "Led 1"(FALSE ("Led 1")) -> ()
            n711 = local write "Led 3"(FALSE ("Led 3")) -> ()
            n712 = local write "Led 2"(TRUE ("Led 2")) -> ()
            n713 = local write "Led 4"(FALSE ("Led 4")) -> ()
            n714 = local write "Led 5"(FALSE ("Led 5")) -> ()
          }
          frame 10 {
            n715 = Boolean To (0,1)(Boolean=FALSE) -> (0, 1=w770:i16)
            n716 = Boolean To (0,1)(Boolean=FALSE) -> (0, 1=w768:i16)
            n717 = Boolean To (0,1)(Boolean=FALSE) -> (0, 1=w769:i16)
            n718 = Boolean To (0,1)(Boolean=TRUE) -> (0, 1=w767:i16)
            n719 = Boolean To (0,1)(Boolean=FALSE) -> (0, 1=w766:i16)
            n720 = local write "Pin2"(w770) -> ()
            n721 = local write "Pin4"(w768) -> ()
            n722 = local write "Pin5"(w767) -> ()
            n723 = local write "Pin3"(w769) -> ()
            n724 = local write "Pin6"(w766) -> ()
            n725 = Wait (ms)(milliseconds to wait=u32 3000 ("millisecond timer value")) -> ()  [unwired: 1 out]
            n726 = local write "Led 1"(FALSE ("Led 1")) -> ()
            n727 = local write "Led 3"(FALSE ("Led 3")) -> ()
            n728 = local write "Led 2"(FALSE ("Led 2")) -> ()
            n729 = local write "Led 4"(TRUE ("Led 4")) -> ()
            n730 = local write "Led 5"(FALSE ("Led 5")) -> ()
          }
          frame 11 {
            n731 = Boolean To (0,1)(Boolean=TRUE) -> (0, 1=w787:i16)
            n732 = Boolean To (0,1)(Boolean=FALSE) -> (0, 1=w785:i16)
            n733 = Boolean To (0,1)(Boolean=FALSE) -> (0, 1=w786:i16)
            n734 = Boolean To (0,1)(Boolean=FALSE) -> (0, 1=w784:i16)
            n735 = Boolean To (0,1)(Boolean=FALSE) -> (0, 1=w783:i16)
            n736 = Wait (ms)(milliseconds to wait=u32 3000 ("millisecond timer value")) -> ()  [unwired: 1 out]
            n737 = local write "Pin2"(w787) -> ()
            n738 = local write "Pin4"(w785) -> ()
            n739 = local write "Pin5"(w784) -> ()
            n740 = local write "Pin3"(w786) -> ()
            n741 = local write "Pin6"(w783) -> ()
            n742 = local write "Contenido"(-1.0 ("Contenido")) -> ()
            n743 = local write "Led 1"(TRUE ("Led 1")) -> ()
            n744 = local write "Led 3"(FALSE ("Led 3")) -> ()
            n745 = local write "Led 2"(FALSE ("Led 2")) -> ()
            n746 = local write "Led 4"(FALSE ("Led 4")) -> ()
            n747 = local write "Led 5"(FALSE ("Led 5")) -> ()
          }
        }
      }
    }
    n748 = call-poly <vilib>:"Digital Read.vi"("Error In"=w36, "DI Channel"=u8 3, "LINX Resource"=w45) -> ("Error Out"=w35:errorcluster, "LINX Resource"=w44:T1)  [unwired: 6 in, 1 out]
    n749 = local read "Led 2"() -> (w25:bool)
    n750 = local write "Pin3"(w28) -> ()
    n751 = call-poly <vilib>:"Digital Write.vi"("Error In"=w35, "Output Value"=w25, "DO Channel"=w28, "LINX Resource"=w44) -> ("Error Out"=w34:errorcluster, "LINX Resource"=w43:T1)  [unwired: 6 in]
    n752 = call-poly <vilib>:"Digital Read.vi"("Error In"=w34, "DI Channel"=u8 4, "LINX Resource"=w43) -> ("Error Out"=w33:errorcluster, "LINX Resource"=w42:T1)  [unwired: 6 in, 1 out]
    n753 = local read "Led 3"() -> (w24:bool)
    n754 = local write "Pin4"(w23) -> ()
    n755 = call-poly <vilib>:"Digital Write.vi"("Error In"=w33, "Output Value"=w24, "DO Channel"=w23, "LINX Resource"=w42) -> ("Error Out"=w32:errorcluster, "LINX Resource"=w41:T1)  [unwired: 6 in]
    n756 = call-poly <vilib>:"Digital Read.vi"("Error In"=w32, "DI Channel"=u8 5, "LINX Resource"=w41) -> ("Error Out"=w31:errorcluster, "LINX Resource"=w40:T1)  [unwired: 6 in, 1 out]
    n757 = local write "Pin5"(w22) -> ()
    n758 = local read "Led 4"() -> (w21:bool)
    n759 = call-poly <vilib>:"Digital Write.vi"("Error In"=w31, "Output Value"=w21, "DO Channel"=w22, "LINX Resource"=w40) -> ("Error Out"=w30:errorcluster, "LINX Resource"=w39:T1)  [unwired: 6 in]
    n760 = call-poly <vilib>:"Digital Read.vi"("Error In"=w30, "DI Channel"=u8 6, "LINX Resource"=w39) -> ("Error Out"=w29:errorcluster, "LINX Resource"=w38:T1)  [unwired: 6 in, 1 out]
    n761 = local write "Pin6"(w19) -> ()
    n762 = local read "Led 5"() -> (w20:bool)
    n763 = call-poly <vilib>:"Digital Write.vi"("Error In"=w29, "Output Value"=w20, "DO Channel"=w19, "LINX Resource"=w38) -> ("Error Out"=w17:errorcluster, "LINX Resource"=w18:T1)  [unwired: 6 in]
  }
  n764 = call <vilib>:"Close.vi"("Error In"=w3, "LINX Resource"=w4) -> ("Error Out"=w11:errorcluster)  [unwired: 9 in]
  n765 = call <vilib>:"Simple Error Handler.vi"("error in (no error)"=w11) -> ()  [unwired: 4 in, 5 out]
  "Contenido" <- 0.0 ("Contenido")
  "Pin2" <- 0.0 ("Pin2")
  "Pin3" <- 0.0 ("Pin3")
  "Pin4" <- 0.0 ("Pin4")
  "Pin5" <- 0.0 ("Pin5")
  "Pin6" <- 0.0 ("Pin6")
